vi "Generador_Posiciones_Minas.vi"(1 "Num_Columnas":dbl, 2 "Num_Filas":dbl, 3 "Num_Minas":dbl) -> (0 "Posiciones_Minas":string[](array[string]))   [LabVIEW 2019]
doc: "Parametros: -----------------------------------------\n\n'Num_Minas': Corresponde al número de minas cuyas posiciones (x,y) seran generadas aleatoriamente, este número no debe superar la cantidad de espacios disponibles en el tablero.\n\n'Num_Filas': corresponde al número total de filas que contiene el tablero.\n\n'Num_Columnas': corresponde al número total de columnas que contiene el tablero.\n\nRetorna: -------------------------------------------------------\n\n'Posiciones_Minas': retorna una lista con cadenas 'x,y' donde x e y corresponden a la posicion de la mina en el tablero."
uses:
  <vilib>/numeric/Random Number (Range) DBL.vi
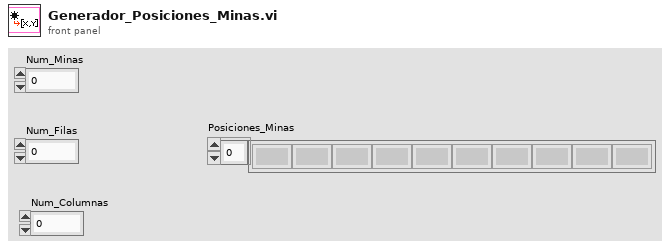
[diagram p1: front panel]
types:
  T1 = enum16{"Generar_posicion_aleatoria", "Validar_elemento_no_repetido", "Agregar_nuevo_item"}
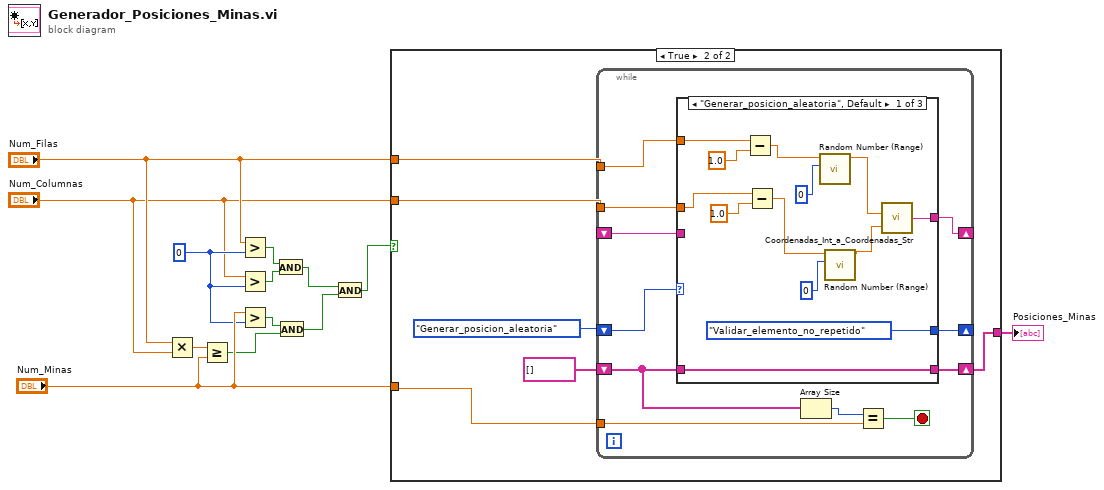
[diagram p0: block diagram]
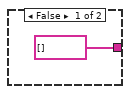
[diagram p2: hidden frame]
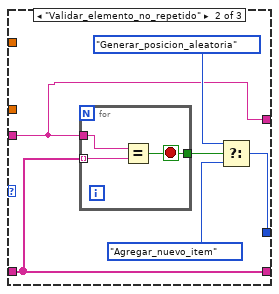
[diagram p3: hidden frame]
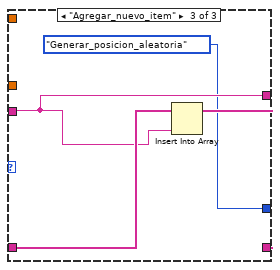
[diagram p4: hidden frame]
diagram:
  w2 = 0
  n1 = Multiply(x="Num_Filas", y="Num_Columnas") -> (x*y=w7:dbl)
  n2 = Greater Or Equal?(x=w7, y="Num_Minas") -> (x >= y?=w4:bool)
  n3 = Greater?(x="Num_Filas", y=w2) -> (0:w11:bool)
  n4 = Greater?(x="Num_Columnas", y=w2) -> (0:w12:bool)
  n5 = Greater?(x="Num_Minas", y=w2) -> (0:w5:bool)
  n6 = And(x=w11, y=w12) -> (x .and. y?=w10:bool)
  n7 = And(x=w5, y=w4) -> (x .and. y?=w3:bool)
  n8 = And(x=w10, y=w3) -> (x .and. y?=w9:bool)
  n9 = case shown="True" w9 {
    tunnel: "Num_Filas" -> [_ w20]
    tunnel: "Num_Columnas" -> [_ w19]
    tunnel: "Num_Minas" -> [_ w15]
    tunnel: [string[] [] ("Array") w16] -> w13
    frame False {
    }
    frame True {
      n10 = while {
        tunnel: w20 -> [w31]
        tunnel: w19 -> [w30]
        shift-right: [w29] -> _
        shift-left: _ -> [w28]
        shift-right: [w27] -> _
        shift-left: T1."Generar_posicion_aleatoria" ("Tareas") -> [w25]
        shift-right: [w26] -> w16
        shift-left: string[] [] ("Array") -> [w24]
        tunnel: w15 -> [w22]
        stop <- w21 stop-if-true
        n11 = case shown="\"Generar_posicion_aleatoria\", Default" w25 {
          tunnel: w31 -> [w42 _ _]
          tunnel: w30 -> [w39 _ _]
          tunnel: [w34 w45 w55] -> w29
          tunnel: w28 -> [_ w45 w55]
          tunnel: [T1."Validar_elemento_no_repetido" ("Tareas") w47 T1."Generar_posicion_aleatoria" ("Tareas")] -> w27
          tunnel: [w35 w46 w57] -> w26
          tunnel: w24 -> [w35 w46 w56]
          frame "Generar_posicion_aleatoria", Default {
            n12 = Subtract(x=w42, y=1.0) -> (x-y=w38:dbl)
            n13 = Subtract(x=w39, y=1.0) -> (x-y=w37:dbl)
            n14 = call-poly <vilib>:"Random Number (Range).vi"("lower bound (0)"=u64 0, "upper bound (100)"=w38) -> ("number"=w33:dbl)  [unwired: 9 in]
            n15 = call-poly <vilib>:"Random Number (Range).vi"("lower bound (0)"=u64 0, "upper bound (100)"=w37) -> ("number"=w32:dbl)  [unwired: 9 in]
            n16 = call "Coordenadas_Int_a_Coordenadas_Str.vi"("Columna"=w32, "Fila"=w33) -> ("Posicion_str"=w34:string)
          }
          frame "Validar_elemento_no_repetido" {
            n17 = for {
              tunnel: w45 -> [w53]
              tunnel: [w52] -> w50
              tunnel: w46 -> [w51] mode=indexing
              stop <- w52 stop-if-true
              n18 = Equal?(x=w53, y=w51) -> (x = y?=w52:bool)
            }
            n19 = Select(t=T1."Generar_posicion_aleatoria" ("Tareas"), s=w50, f=T1."Agregar_nuevo_item" ("Tareas")) -> (s? t:f=w47:T1)
          }
          frame "Agregar_nuevo_item" {
            n20 = Insert Into Array(array=w56, new element=w55) -> (w57:string[])  [unwired: 1 in]
          }
        }
        n21 = Array Size(array=w24) -> (size(s)=w23:i32)
        n22 = Equal?(x=w23, y=w22) -> (x = y?=w21:bool)
      }
    }
  }
  "Posiciones_Minas" <- w13
